vi "CheckCore.vi"(8 "error in (no error)":errorcluster, 9 "# of Refs":i32, 10 "References":refnum<vi>[](array[refnum]), 11 "Blacklist in":refnum<class "Blacklist.lvclass">) -> (0 "error out":errorcluster, 1 "Reject?":bool, 2 "dup References":refnum<vi>[](array[refnum]), 3 "Blacklist out":refnum<class "Blacklist.lvclass">)   [LabVIEW 2014, in "BuildSecurity.lvlib" / "Blacklist.lvclass"]
doc: "Base functionality for determining if an item is blacklisted. Child classes must override this to implement class-specific blacklist processing."
uses:
  Blacklist.lvclass
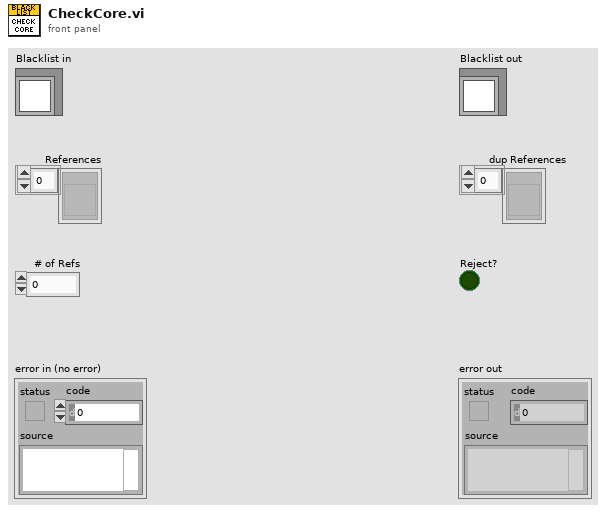
[diagram p1: front panel]
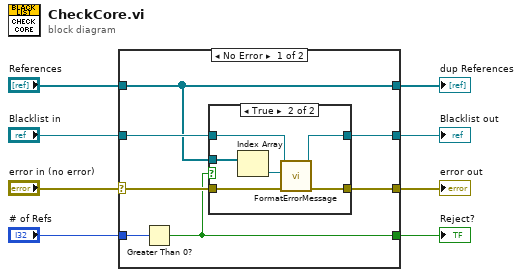
[diagram p0: block diagram]
diagram:
  n1 = case shown="No Error" "error in (no error)" {
    selector: "error in (no error)" -> [w11 w26]
    tunnel: [w9 w26] -> w7
    tunnel: [w14 w25] -> w5
    tunnel: "Blacklist in" -> [w15 w25]
    tunnel: "References" -> [w12 w24]
    tunnel: [w12 w24] -> w3
    tunnel: "# of Refs" -> [w13 _]
    tunnel: [w10 _] -> w1
    frame No Error {
      n2 = Greater Than 0?(x=w13) -> (x > 0?=w10:bool)
      n3 = case shown="True" w10 {
        tunnel: w15 -> [w17 w19]
        tunnel: [w17 w18] -> w14
        tunnel: w12 -> [_ w23]
        tunnel: w11 -> [w16 w21]
        tunnel: [w16 w20] -> w9
        frame False {
        }
        frame True {
          n4 = Index Array(array=w23) -> (element=w22:refnum<vi>)  [unwired: 1 in]
          n5 = call-dynamic "FormatErrorMessage.vi"("error in (no error)"=w21, "GObj Refnum"=w22, "Blacklist in"=w19) -> ("error out"=w20:errorcluster, "Blacklist out"=w18:refnum<class "Blacklist.lvclass">)  [unwired: 6 in, 1 out]
        }
      }
    }
    frame Error {
    }
  }
  "error out" <- w7
  "Blacklist out" <- w5
  "dup References" <- w3
  "Reject?" <- w1
